vi "Main.vi"(11 "Module Admin":refnum<class "Delacor_lib_QMH_Module Admin.lvclass">) -> ()   [LabVIEW 2019, in "Base de datos.lvlib"]
doc: "This template is based off of the Queued Message Handler design pattern and the Queued Message Handler project template that ships with LabVIEW.\n\nThe main difference is that the queue is private to this module and communication between modules is performed via Broadcast and Request events.\n\nRequest events are wrapped in public API methods and are handled in the Event Handling Loop (EHL) of this VI. Any module can register for Broadcast events sent by this module. The EHL generates messages based on user interface actions.\n\nThe Message Handling Loop (MHL) processes messages generated by the EHL, or by other messages. The messages are string values, so new messages can be added easily to the Message Cases case structure in the MHL. Each message cluster can also provide an optional value for Message Data, which is a variant that can be converted to whatever message-specific data is required.\n_____\nBased on Delacor QMH Project Template 5.0.0.82."
uses:
  Base de datos.lvlib
  <vilib>/Delacor/Delacor QMH/Libraries/Module Admin_class/Delacor_lib_QMH_Module Admin.lvclass
  Module Data--cluster.ctl
  Stop Argument--cluster.ctl
  <vilib>/Delacor/Delacor QMH/Libraries/Message Queue_class/Delacor_lib_QMH_Message Queue.lvclass/Delacor_lib_QMH_Message Queue.ctl
  <vilib>/Delacor/Delacor QMH/Libraries/Module Admin_class/Delacor_lib_QMH_Module Admin.lvclass/Delacor_lib_QMH_Module Admin.ctl
  <vilib>/Utility/miscctls.llb/LVPointTypeDef.ctl
  <vilib>/Delacor/Delacor QMH/Libraries/Message Queue_class/Delacor_lib_QMH_Enqueue Message (Single).vi
  <vilib>/Delacor/Delacor QMH/Libraries/Module Admin_class/Delacor_lib_QMH_Get External Launch.vi
  <vilib>/Utility/error.llb/Error Cluster From Error Code.vi
  <vilib>/ErrorRing/Error Ring.xnode
  <vilib>/Delacor/Delacor QMH/Libraries/Message Queue_class/Delacor_lib_QMH_Message Queue.lvclass
panel:
  out "error out":errorcluster
  out "Status":string
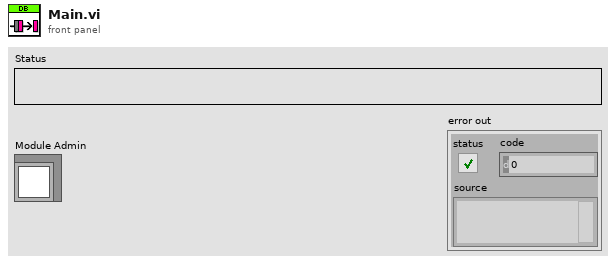
[diagram p1: front panel]
types:
  T1 = typedef "Base de datos.lvlib/Request Events--cluster.ctl" = cluster{"Stop Module":refnum<user-event>, "Show Panel":refnum<user-event>, "Hide Panel":refnum<user-event>, "Get Module Execution Status":refnum<user-event>, "Show Diagram":refnum<user-event>, "Config Database":refnum<user-event>, "Iniciar base de datos":refnum<user-event>, "Parar Base de datos":refnum<user-event>, "Escribir":refnum<user-event>, "Datos de analisis":refnum<user-event>}
  T2 = typedef "Base de datos.lvlib/Module Data--cluster.ctl" = cluster{"Status":string}
  T3 = enum32{"invalid lock state", "Not Locked", "Locked (No Password)", "Password-protected"}
  T4 = typedef "Base de datos.lvlib/Stop Argument--cluster.ctl" = cluster{"Origin":string, "Exit via Stop Module Req?":bool, "Wait for Module to stop?":bool}
  T5 = typedef "LVPointTypeDef.ctl" = cluster{"Horizontal":i16, "Vertical":i16}
  T6 = enum32{"Invalid", "Standard", "Closed", "Hidden", "Minimized", "Maximized"}
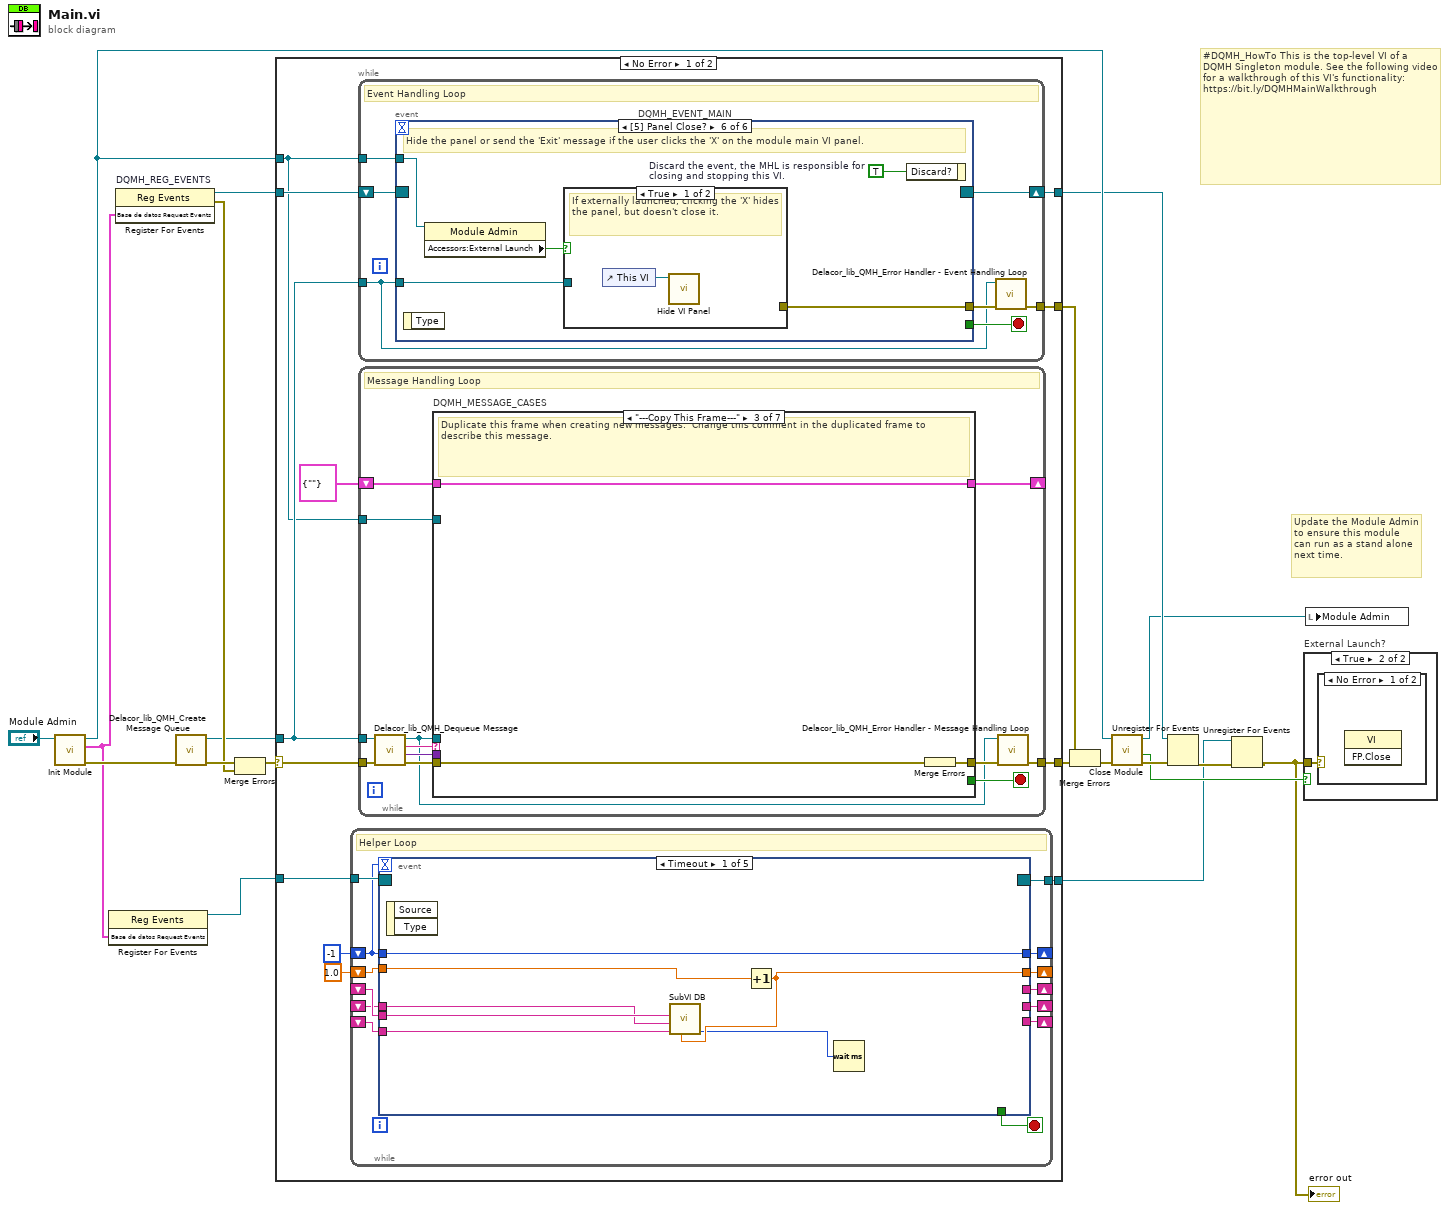
[diagram p0: block diagram]
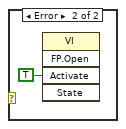
[diagram p3: hidden frame]
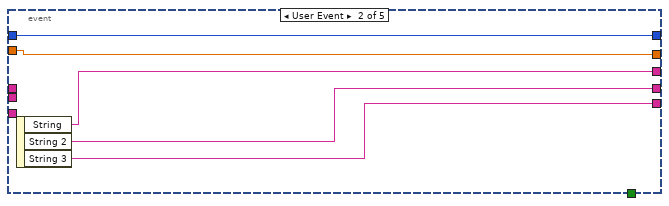
[diagram p4: hidden frame]
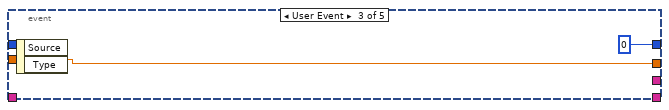
[diagram p5: hidden frame]
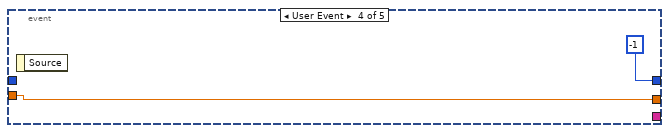
[diagram p6: hidden frame]
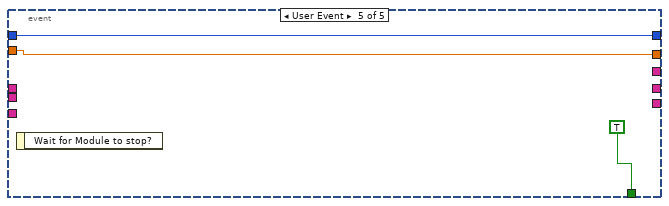
[diagram p7: hidden frame]
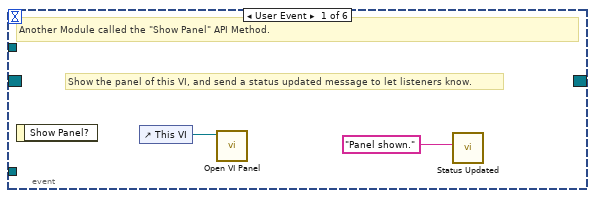
[diagram p8: hidden frame]
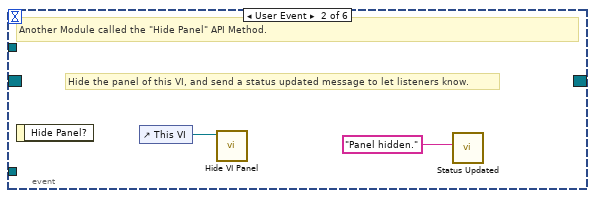
[diagram p9: hidden frame]
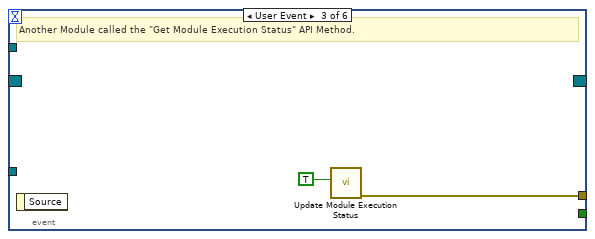
[diagram p10: hidden frame]
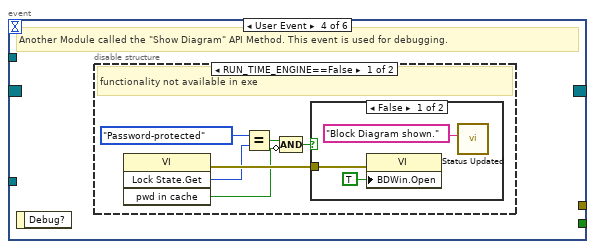
[diagram p11: hidden frame]
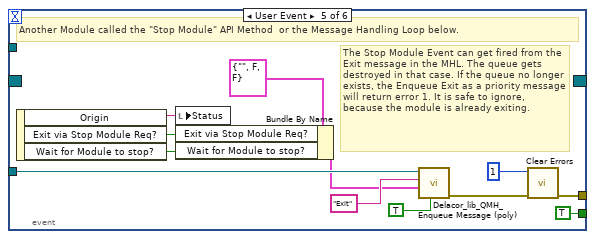
[diagram p14: hidden frame]
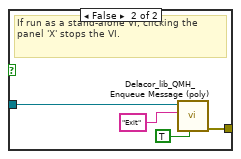
[diagram p15: hidden frame]
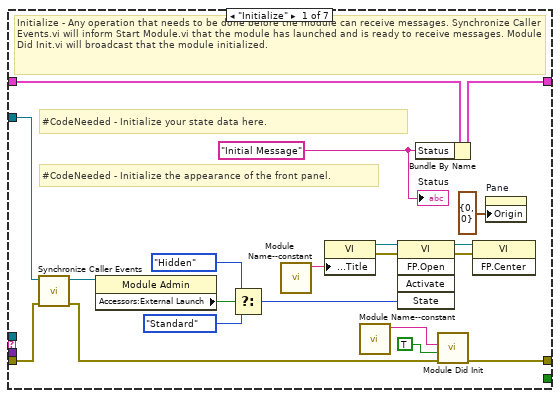
[diagram p16: hidden frame]
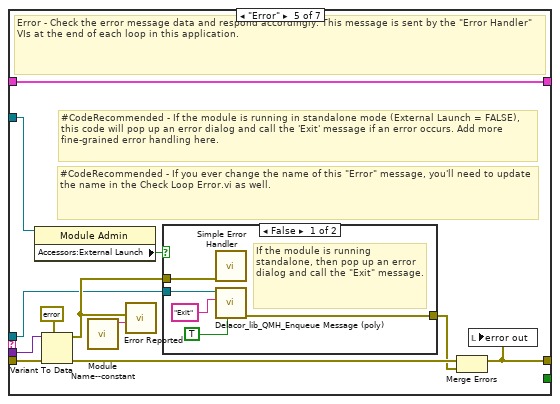
[diagram p19: hidden frame]
diagram:
  # "#DQMH_HowTo This is the top-level VI of a DQMH Singleton module. See the following video for a walkthrough of this VI's functionality: https://bit.ly/DQMHMainWalkthrough"
  # "Update the Module Admin to ensure this module can run as a stand alone next time."
  n1 = call "Init Module.vi"("Singleton Module Admin in"="Module Admin") -> ("error out"=w19:errorcluster, "Base de datos Request Events"=w5:T1, "Singleton Module Admin out"=w12:refnum<class "Delacor_lib_QMH_Module Admin.lvclass">)  [unwired: 8 in]
  n2 = register-events(w5) -> (reference out=w4:refnum<event-registration>)  [unwired: 2 in, 1 out]
  n3 = register-events "DQMH_REG_EVENTS"(w5) -> (reference out=w10:refnum<event-registration>, error out=w13:errorcluster)  [unwired: 2 in]
  n4 = call <vilib>:"Delacor_lib_QMH_Create Message Queue.vi"("error in (no error)"=w19) -> ("error out"=w15:errorcluster, "Message Queue"=w9:refnum<class "Delacor_lib_QMH_Message Queue.lvclass">)  [unwired: 9 in]
  n5 = Merge Errors(w15, w13) -> (w14:errorcluster)
  n6 = case shown="No Error" w14 {
    selector: w14 -> [w30 w197]
    tunnel: [w32 w196] -> w20
    tunnel: [w29 w202] -> w11
    tunnel: w10 -> [w27 w202]
    tunnel: w9 -> [w26 w195]
    tunnel: [w31 _] -> w17
    tunnel: w12 -> [w25 w198]
    tunnel: w4 -> [w24 w194]
    tunnel: [w23 w194] -> w1
    frame No Error {
      n7 = while {
        tunnel: w24 -> [w45]
        tunnel: [w44] -> w23
        shift-right: [w42] -> _
        shift-left: -1 -> [w41]
        shift-right: [w40] -> _
        shift-left: _ -> [w37]
        shift-right: [w39] -> _
        shift-left: _ -> [w36]
        shift-right: [w38] -> _
        shift-left: _ -> [w35]
        shift-right: [w34] -> _
        shift-left: 1.0 -> [w33]
        stop <- w43 stop-if-true
        # "Helper Loop"
        n8 = event shown="[0] Timeout" {
          selector: w45 -> [_ _ _ _ _]
          dyn-events: [_ _ _ _ _] -> w44
          timeout: w41 -> [_ _ _ _ _]
          tunnel: [_ _ _ _ TRUE] -> w43
          tunnel: [w52 w54 0 -1 w62] -> w42
          tunnel: w41 -> [w52 w54 _ _ w62]
          tunnel: [_ w57 _ _ _] -> w40
          tunnel: [_ w56 _ _ _] -> w39
          tunnel: [_ w55 _ _ _] -> w38
          tunnel: w37 -> [w51 _ _ _ _]
          tunnel: w36 -> [w50 _ _ _ _]
          tunnel: w35 -> [w49 _ _ _ _]
          tunnel: [w48 w53 w58 w60 w63] -> w34
          tunnel: w33 -> [w47 w53 w58 w60 w63]
          event Timeout {
            n9 = event-data() -> ()  [unwired: 1 in, 2 out]
            n10 = Increment(x=w47) -> (x+1=w48:dbl)
            n11 = call "SubVI DB.vi"("Numeric"=w48, "Empresa"=w49, "Area"=w50, "Nombre"=w51) -> ("Numeric 2"=w46:i32)  [unwired: 7 in]
            n12 = Wait (ms)(milliseconds to wait=w46) -> ()  [unwired: 1 out]
          }
          event User Event {
            n13 = event-data() -> ("String"=w57:string, "String 2"=w56:string, "String 3"=w55:string)  [unwired: 1 in]
          }
          event User Event {
            n14 = event-data() -> ()  [unwired: 1 in, 2 out]
          }
          event User Event {
            n15 = event-data() -> ()  [unwired: 1 in, 1 out]
          }
          event User Event {
            n16 = event-data() -> ()  [unwired: 1 in, 1 out]
          }
        }
      }
      n17 = while {
        tunnel: w26 -> [w65]
        shift-right: [w68] -> w29
        shift-left: w27 -> [w69]
        tunnel: [w70] -> w31
        tunnel: w25 -> [w66]
        stop <- w67 stop-if-true
        # "Event Handling Loop"
        n18 = event "DQMH_EVENT_MAIN" shown="[5] Panel Close?" {
          selector: w69 -> [_ _ _ _ _ _]
          dyn-events: [_ _ _ _ _ _] -> w68
          timeout: _ -> [_ _ _ _ _ _]
          tunnel: [_ _ _ _ TRUE ("Discard?") _] -> w67
          tunnel: w65 -> [_ _ _ _ w94 w101]
          tunnel: [_ _ w77 _ w97 w103] -> w71
          tunnel: w66 -> [_ _ _ _ _ w100]
          event User Event {
            # "Show the panel of this VI, and send a status updated message to let listeners know."
            # "Another Module called the \"Show Panel\" API Method."
            n19 = event-data() -> ()  [unwired: 1 in, 1 out]
            n20 = control-ref of="This VI"() -> (w73:refnum<vi>)
            n21 = call "Open VI Panel.vi"("VI"=w73) -> ()  [unwired: 10 in, 1 out]
            n22 = call "Status Updated.vi"("Status"="Panel shown." ("format string")) -> ()  [unwired: 10 in, 1 out]
          }
          event User Event {
            # "Hide the panel of this VI, and send a status updated message to let listeners know."
            # "Another Module called the \"Hide Panel\" API Method."
            n23 = event-data() -> ()  [unwired: 1 in, 1 out]
            n24 = control-ref of="This VI"() -> (w75:refnum<vi>)
            n25 = call "Hide VI Panel.vi"("VI"=w75) -> ()  [unwired: 10 in, 1 out]
            n26 = call "Status Updated.vi"("Status"="Panel hidden." ("format string")) -> ()  [unwired: 10 in, 1 out]
          }
          event User Event {
            # "Another Module called the \"Get Module Execution Status\" API Method."
            n27 = event-data() -> ()  [unwired: 1 in, 1 out]
            n28 = call "Update Module Execution Status.vi"("Running?"=TRUE) -> ("error out"=w77:errorcluster)  [unwired: 10 in]
          }
          event User Event {
            # "Another Module called the \"Show Diagram\" API Method. This event is used for debugging."
            n29 = event-data() -> ()  [unwired: 1 in, 1 out]
            n30 = disable-structure shown="RUN_TIME_ENGINE==False" {
              frame condition #0 (active) {
                # "functionality not available in exe"
                n31 = invoke class="VI" method="Lock State.Get"() -> (error out=w83:errorcluster, "Get Lock State"=w82:T3, "pwd in cache"=w79:bool)  [unwired: 4 in, 1 out]
                n32 = Equal?(x=T3."Password-protected", y=w82) -> (x = y?=w80:bool)
                n33 = Compound Arithmetic op=AND(w80, invert w79) -> (w78:bool)
                n34 = case shown="False" w78 {
                  tunnel: w83 -> [w86 _]
                  frame False {
                    n35 = property class="VI"(error in=w86, "BDWin.Open"=TRUE ("Block Diagram Window:Open")) -> ()  [unwired: 1 in, 2 out]
                    n36 = call "Status Updated.vi"("Status"="Block Diagram shown." ("format string")) -> ()  [unwired: 10 in, 1 out]
                  }
                  frame True {
                    # "Password-protected VI, and the password is not in the cache. Do not show the diagram."
                  }
                }
              }
              frame condition #1 {
              }
            }
          }
          event User Event {
            # "The Stop Module Event can get fired from the Exit message in the MHL. The queue gets destroyed in that case. If the queue no longer exists, the Enqueue Exit as a priority message will return error 1. It is safe to ignore, because the module is already exiting."
            # "Another Module called the \"Stop Module\" API Method  or the Message Handling Loop below."
            n37 = event-data() -> ("Origin"=w93:string, "Exit via Stop Module Req?"=w89:bool, "Wait for Module to stop?"=w88:bool)  [unwired: 1 in]
            n38 = local write "Status"(w93) -> ()
            n39 = Bundle By Name(cluster=T4 {"Origin"="", "Exit via Stop Module Req?"=FALSE, "Wait for Module to stop?"=FALSE} ("Stop Argument"), "Exit via Stop Module Req?"=w89, "Wait for Module to stop?"=w88) -> (w87:T4)
            n40 = call-poly <vilib>:"Delacor_lib_QMH_Enqueue Message (poly).vi"("Priority Message? (F)"=TRUE, "Message Data"=w87, "Message"="Exit", "Message Queue in"=w94) -> ("error out"=w98:errorcluster)  [unwired: 6 in, 1 out]
            n41 = call <vilib>:"Clear Errors.vi"("error in (no error)"=w98, "specific error code to clear (0: all)"=1) -> ("error out"=w97:errorcluster)  [unwired: 4 in, 1 out]
          }
          event Panel Close? {
            w102 = TRUE  # Discard the event, the MHL is responsible for closing and stopping this VI.
            # "Hide the panel or send the 'Exit' message if the user clicks the 'X' on the module main VI panel."
            n42 = event-data() -> ()  [unwired: 1 in, 1 out]
            n43 = property class="Module Admin"(reference=w100) -> ("Accessors:External Launch"=w99:bool)  [unwired: 1 in, 2 out]
            n44 = case shown="True" w99 {
              tunnel: w101 -> [_ w107]
              tunnel: [_ w108] -> w103
              frame True {
                # "If externally launched, clicking the 'X' hides the panel, but doesn't close it."
                n45 = control-ref of="This VI"() -> (w104:refnum<vi>)
                n46 = call "Hide VI Panel.vi"("VI"=w104) -> ()  [unwired: 10 in, 1 out]
              }
              frame False {
                # "If run as a stand-alone VI, clicking the panel 'X' stops the VI."
                n47 = call-poly <vilib>:"Delacor_lib_QMH_Enqueue Message (poly).vi"("Priority Message? (F)"=TRUE, "Message"="Exit", "Message Queue in"=w107) -> ("error out"=w108:errorcluster)  [unwired: 7 in, 1 out]
              }
            }
            n48 = event-data("Discard?"=w102) -> ()  [unwired: 1 in, 1 out]
          }
        }
        n49 = call-dynamic "Delacor_lib_QMH_Error Handler - Event Handling Loop.vi"("error in (no error)"=w71, "Message Queue in"=w65) -> ("dup error in"=w70:errorcluster)  [unwired: 8 in, 1 out]
      }
      n50 = while {
        tunnel: w26 -> [w111]
        shift-right: [w115] -> _
        shift-left: T2 {"Status"=""} ("Data Cluster") -> [w116]
        tunnel: w30 -> [w119]
        tunnel: [w117] -> w32
        tunnel: w25 -> [w109]
        stop <- w114 stop-if-true
        # "Message Handling Loop"
        n51 = call-dynamic "Delacor_lib_QMH_Dequeue Message.vi"("error in (no error)"=w119, "Message Queue in"=w111) -> ("error out"=w118:errorcluster, "Message Data"=w112:variant, "Message"=w113:string, "Message Queue out"=w110:refnum<class "Delacor_lib_QMH_Message Queue.lvclass">)  [unwired: 6 in]
        n52 = case "DQMH_MESSAGE_CASES" shown="\"---Copy This Frame---\"" w113 {
          selector: w113 -> [_ _ _ _ _ _ w181]
          tunnel: w110 -> [_ _ _ _ w151 w173 _]
          tunnel: w118 -> [w138 w142 w145 w147 w158 w179 w183]
          tunnel: [w136 w142 w144 w147 w154 w176 w184] -> w120
          tunnel: w116 -> [w127 w141 w143 w146 w153 w172 w182]
          tunnel: [w126 w141 w143 w146 w153 w172 w182] -> w115
          tunnel: [_ _ _ _ _ w171 _] -> w114
          tunnel: w112 -> [_ _ _ _ w152 w170 _]
          tunnel: w109 -> [w128 _ _ _ w150 w165 _]
          frame "Initialize" {
            w121 = "Initial Message" ("Initial Message")
            # "#CodeNeeded - Initialize the appearance of the front panel."
            # "#CodeNeeded - Initialize your state data here."
            # "Initialize - Any operation that needs to be done before the module can receive messages. Synchronize Caller Events.vi will inform Start Module.vi that the module has launched and is ready to receive messages. Module Did Init.vi will broadcast that the module initialized."
            n53 = call "Synchronize Caller Events.vi"("error in (no error)"=w138, "Singleton Module Admin in"=w128) -> ("error out"=w137:errorcluster, "Singleton Module Admin out"=w123:refnum<class "Delacor_lib_QMH_Module Admin.lvclass">)  [unwired: 8 in]
            n54 = property class="Module Admin"(reference=w123) -> ("Accessors:External Launch"=w132:bool)  [unwired: 1 in, 2 out]
            n55 = Select(t=T6."Hidden" ("State"), s=w132, f=T6."Standard" ("State")) -> (s? t:f=w129:T6)
            n56 = call "Module Name--constant.vi"() -> ("Module Name"=w135:string)  [unwired: 11 in]
            n57 = property class="VI"("Front Panel.Title"=w135) -> (reference out=w134:refnum<vi>, error out=w140:errorcluster)  [unwired: 2 in]
            n58 = call "Module Name--constant.vi"() -> ("Module Name"=w124:string)  [unwired: 11 in]
            n59 = invoke class="VI" method="FP.Open"(reference=w134, error in=w140, "State"=w129) -> (reference out=w133:refnum<vi>, error out=w139:errorcluster)  [unwired: 2 in, 3 out]
            n60 = Bundle By Name(cluster=w127, "Status"=w121) -> (w126:T2)
            n61 = call "Module Did Init.vi"("error in (no error)"=w137, "Initialized?"=TRUE, "Origin"=w124) -> ("error out"=w136:errorcluster)  [unwired: 8 in]
            n62 = invoke class="VI" method="FP.Center"(reference=w133, error in=w139) -> ()  [unwired: 1 in, 3 out]
            n63 = property on="Pane" class="Pane"("Origin"=T5 {"Horizontal"=0, "Vertical"=0}) -> ()  [unwired: 2 in, 2 out]
            "Status" <- w121
          }
          frame "--- Module Specific ---" {
            # "Separator -- The following cases handle messages specific to this Module."
          }
          frame "---Copy This Frame---" {
            # "Duplicate this frame when creating new messages.  Change this comment in the duplicated frame to describe this message."
            n64 = Merge Errors(w145) -> (w144:errorcluster)
          }
          frame "--- Exit and Error Handling---" {
            # "Separator - The following cases handle errors and exit messages."
          }
          frame "Error" {
            # "#CodeRecommended - If you ever change the name of this \"Error\" message, you'll need to update the name in the Check Loop Error.vi as well."
            # "#CodeRecommended - If the module is running in standalone mode (External Launch = FALSE), this code will pop up an error dialog and call the 'Exit' message if an error occurs. Add more fine-grained error handling here."
            # "Error - Check the error message data and respond accordingly. This message is sent by the \"Error Handler\" VIs at the end of each loop in this application."
            n65 = property class="Module Admin"(reference=w150) -> ("Accessors:External Launch"=w149:bool)  [unwired: 1 in, 2 out]
            n66 = Variant To Data(error in=w158, type=errorcluster {"status"=FALSE, "code"=0, "source"=""} ("error constant"), Variant=w152) -> (data=w159:errorcluster, error out=w156:errorcluster)
            n67 = call "Module Name--constant.vi"() -> ("Module Name"=w148:string)  [unwired: 11 in]
            n68 = call "Error Reported.vi"("Additional Information"=w148, "Error"=w159) -> ()  [unwired: 9 in, 1 out]
            n69 = case shown="False" w149 {
              tunnel: [w164 _] -> w155
              tunnel: w151 -> [w162 _]
              tunnel: w159 -> [w163 _]
              frame False {
                # "If the module is running standalone, then pop up an error dialog and call the \"Exit\" message."
                n70 = call <vilib>:"Simple Error Handler.vi"("error in (no error)"=w163) -> ()  [unwired: 4 in, 5 out]
                n71 = call-poly <vilib>:"Delacor_lib_QMH_Enqueue Message (poly).vi"("Priority Message? (F)"=TRUE, "Message"="Exit", "Message Queue in"=w162) -> ("error out"=w164:errorcluster)  [unwired: 7 in, 1 out]
              }
              frame True {
                # "If the module was launched externally, calling the Error Reported broadcast VI is the only action performed by the \"Error\" message. The module's caller can then process the error appropriately."
              }
            }
            n72 = Merge Errors(w156, w155) -> (w154:errorcluster)
            n73 = local write "error out"(w154) -> ()
          }
          frame "Exit" {
            w169 = 91  # 91: not all Exit messages will have an argument
            w171 = TRUE  # Stop the VI
            # "Release the message queue reference"
            # "#CodeNeeded - Add any required cleanup code here"
            # "Exit - Exit the application."
            n74 = Variant To Data(error in=w179, type=T4 {"Origin"="", "Exit via Stop Module Req?"=FALSE, "Wait for Module to stop?"=FALSE} ("Stop Argument"), Variant=w170) -> (data=w167:T4, error out=w175:errorcluster)
            n75 = call <vilib>:"Clear Errors.vi"("error in (no error)"=w175, "specific error code to clear (0: all)"=w169) -> ("error out"=w178:errorcluster)  [unwired: 4 in, 1 out]
            n76 = control-ref of="This VI"() -> (w166:refnum<vi>)
            n77 = call-dynamic "Delacor_lib_QMH_Release Message Queue.vi"("error in (no error)"=w178, "Message Queue"=w173) -> ("error out"=w177:errorcluster)  [unwired: 9 in]
            n78 = call "Handle Exit.vi"("Stop Argument"=w167, "Admin in"=w165, "VI reference"=w166) -> ("error out"=w174:errorcluster)  [unwired: 7 in, 1 out]
            n79 = Merge Errors(w177, w174) -> (w176:errorcluster)
          }
          frame Default {
            # "'Default' case only runs if there is a message that isn't defined in any of the other cases.  Output a programming error."
            n80 = call "Module Name--constant.vi"() -> ("Module Name"=w180:string)  [unwired: 11 in]
            n81 = xnode "Error Ring"("parameter 0"=w181, "parameter 1"=w180) -> ("error out"=w185:errorcluster)
            n82 = Merge Errors(w183, w185) -> (w184:errorcluster)
          }
        }
        n83 = call-dynamic "Delacor_lib_QMH_Error Handler - Message Handling Loop.vi"("error in (no error)"=w120, "Message Queue in"=w110) -> ("dup error in"=w117:errorcluster)  [unwired: 8 in, 1 out]
      }
    }
    frame Error {
      # "Synchronize Caller Events.vi will inform Start Module.vi that the module has launched and will let the code calling Start Module.vi register for broadcasts and would permit the caller receive the broadcast that an error occurred at launch time."
      n84 = call-dynamic "Delacor_lib_QMH_Release Message Queue.vi"("error in (no error)"=w197, "Message Queue"=w195) -> ("error out"=w196:errorcluster)  [unwired: 9 in]
      n85 = call "Synchronize Caller Events.vi"("Singleton Module Admin in"=w198) -> ("error out"=w203:errorcluster)  [unwired: 9 in, 1 out]
      n86 = call "Module Name--constant.vi"() -> ("Module Name"=w201:string)  [unwired: 11 in]
      n87 = Format Into String(format string="An error occurred during initialization. %s is no longer running.", w201) -> (resulting string=w199:string)  [unwired: 2 in, 1 out]
      n88 = Merge Errors(w196, w203) -> (w204:errorcluster)
      n89 = call "Error Reported.vi"("Additional Information"=w199, "Error"=w204) -> ()  [unwired: 9 in, 1 out]
    }
  }
  n90 = Merge Errors(w17, w20) -> (w16:errorcluster)
  n91 = call "Close Module.vi"("error in (no error)"=w16, "Module Admin in"=w12) -> ("error out"=w18:errorcluster, "External Launch"=w6:bool, "Module Admin out"=w7:refnum<class "Delacor_lib_QMH_Module Admin.lvclass">)  [unwired: 7 in]
  n92 = Unregister For Events(event registration refnum=w11, error in=w18) -> (error out=w2:errorcluster)
  n93 = Unregister For Events(event registration refnum=w1, error in=w2) -> (error out=w3:errorcluster)
  "error out" <- w3
  n94 = case "External Launch?" shown="True" w6 {
    tunnel: w3 -> [_ w205]
    frame False {
    }
    frame True {
      n95 = case shown="No Error" w205 {
        frame No Error {
          n96 = invoke class="VI" method="FP.Close"() -> ()  [unwired: 3 in, 3 out]
        }
        frame Error {
          n97 = invoke class="VI" method="FP.Open"("Activate"=TRUE ("Activate?")) -> ()  [unwired: 4 in, 5 out]
        }
      }
    }
  }
  n98 = local write "Module Admin"(w7) -> ()
